vi "edittest export sequence.vi"(6 "User":T1, 8 "error in (no error)":errorcluster, 10 "Sequence ID":string, 11 "Connection Refnum":T2) -> (0 "error out":errorcluster, 2 "Exported Sequence":string, 3 "Connection Refnum":T2)   [LabVIEW 2011]
uses:
  SI.LIB/ODBC/SQL Controls/Connection Refnum.ctl
  server/database/Users/User Record.ctl
  sequence xml.ctl
  server/database/Sequences/Sequence Record.ctl
  server/database/Steps/Step Record.ctl
  server/database/Fields/Field Record.ctl
  server/database/Fields/Field DataTypes.ctl
  server/database/Fields/Field NextItem.ctl
  server/server lib/Spartan Version.vi
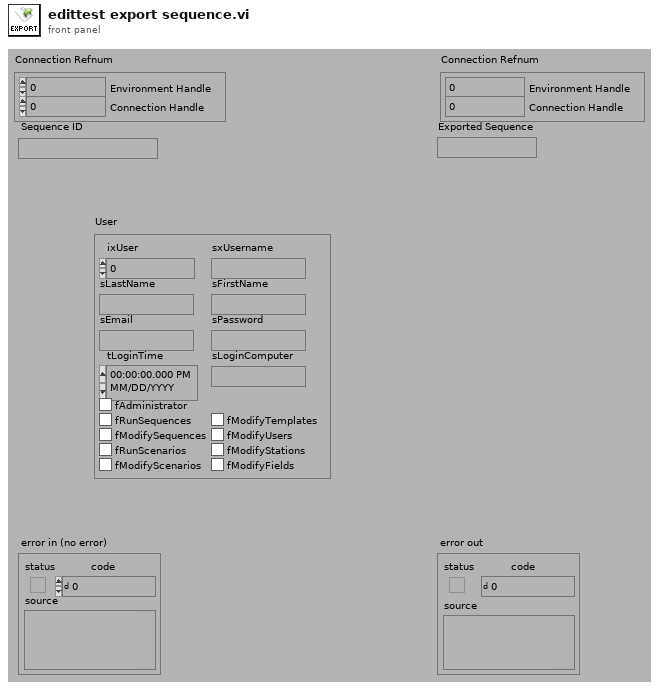
[diagram p1: front panel]
types:
  T1 = typedef "User Record.ctl" = cluster{"ixUser":i32, "sxUsername":string, "sLastName":string, "sFirstName":string, "sEmail":string, "sPassword":string, "tLoginTime":timestamp, "sLoginComputer":string, "fAdministrator":bool, "fRunSequences":bool, "fModifySequences":bool, "fRunScenarios":bool, "fModifyScenarios":bool, "fModifyTemplates":bool, "fModifyUsers":bool, "fModifyStations":bool, "fModifyFields":bool}
  T2 = typedef "Connection Refnum.ctl" = cluster{"Environment Handle":i32, "Connection Handle":i32}
  T3 = typedef "sequence xml.ctl" = cluster{"#attributes":cluster{"Version":string, "Creator":string}, "Sequence":T4, "Steps":T5[], "Fields":T6[]}
  T4 = typedef "Sequence Record.ctl" = cluster{"ixSequence":i32, "sxSequenceId":string, "sDescription":string, "sCreator":string, "tCreationDate":timestamp, "sModifier":string, "tModifiedDate":timestamp, "fApproved":bool, "fSpartanSetsSN":bool, "fOverwriteData":bool, "fStopOnFail":bool, "fDisableQuickMode":bool, "fPartialExecution":bool, "fAutoNextItem":bool, "fDoNotPrintOnFail":bool}
  T5 = typedef "Step Record.ctl" = cluster{"ixStep":i32, "sxSequenceId":string, "sxTestId":string, "iIndex":i32, "iRepeat":i32, "iQuickMode":i32, "sTag":string, "sDatasheetsCSV":string, "bConfiguration":string}
  T6 = typedef "Field Record.ctl" = cluster{"ixField":i32, "iSequenceOrder":i32, "sxFieldId":string, "sxSequenceId":string, "sDisplayName":string, "sValue":string, "sUnits":string, "nDataType":T7, "nNextItem":T8, "fSystem":bool, "fSystemValue":bool, "fRequired":bool, "fSetAtTest":bool, "fTestField":bool, "fDeleted":bool, "fIndexed":bool, "fFreeList":bool}
  T7 = typedef "Field DataTypes.ctl" = enum32{"text", "numeric", "list", "timestamp", "boolean"}
  T8 = typedef "Field NextItem.ctl" = enum32{"Reset", "Retain", "Auto-Increment"}
  T9 = typedef "OGAB Version.ctl" = cluster{"Version":string, "Build Number":u32, "Build Date/Time":dbl}
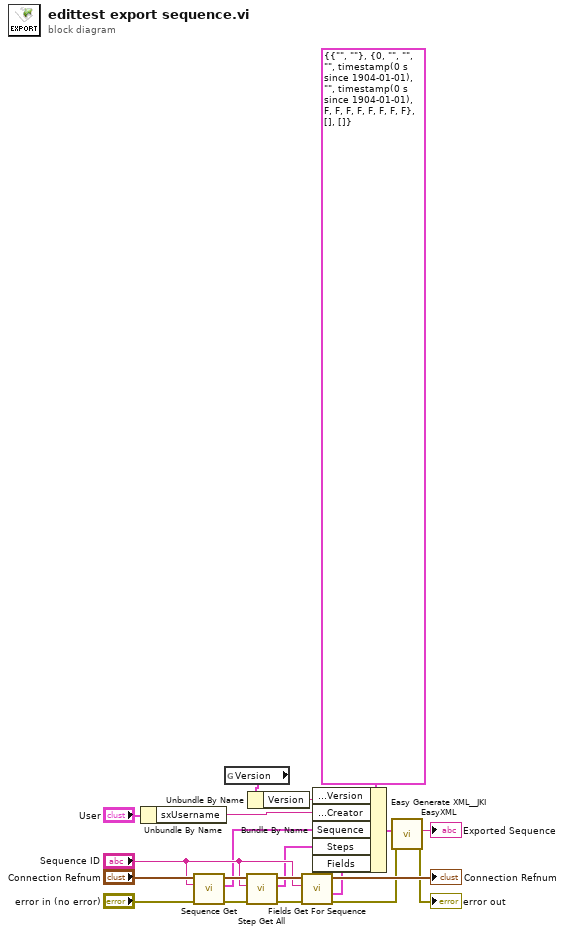
[diagram p0: block diagram]
diagram:
  n1 = Unbundle By Name("User") -> ("sxUsername"=w8:string)
  n2 = call "Sequence Get.vi"("error in (no error)"="error in (no error)", "sxSequenceId (\"\")"="Sequence ID", "Connection Refnum"="Connection Refnum") -> ("error out"=w19:errorcluster, "Sequence Record"=w7:T4, "Connection Refnum"=w16:T2)  [unwired: 6 out]
  n3 = global read "Spartan Version.vi" "Version"() -> (w10:T9)
  n4 = call "Step Get All.vi"("error in (no error)"=w19, "sxSequenceId"="Sequence ID", "Connection Refnum"=w16) -> ("error out"=w17:errorcluster, "Sequence Steps"=w6:T5[], "Connection Refnum"=w15:T2)  [unwired: 1 in, 5 out]
  n5 = Unbundle By Name(w10) -> ("Version"=w9:string)
  n6 = call "Fields Get For Sequence.vi"("error in (no error)"=w17, "sxSequenceId (\"\")"="Sequence ID", "Connection Refnum"=w15) -> ("error out"=w3:errorcluster, "Current Sequence Fields"=w5:T6[], "Connection Refnum"=→"Connection Refnum":T2)  [unwired: 6 out]
  n7 = Bundle By Name(cluster=T3 {"#attributes"={"Version"="", "Creator"=""}, "Sequence"={"ixSequence"=0, "sxSequenceId"="", "sDescription"="", "sCreator"="", "tCreationDate"=timestamp(0 s since 1904-01-01), "sModifier"="", "tModifiedDate"=timestamp(0 s since 1904-01-01), "fApproved"=FALSE, "fSpartanSetsSN"=FALSE, "fOverwriteData"=FALSE, "fStopOnFail"=FALSE, "fDisableQuickMode"=FALSE, "fPartialExecution"=FALSE, "fAutoNextItem"=FALSE, "fDoNotPrintOnFail"=FALSE}, "Steps"=[], "Fields"=[]} ("Sequence"), "#attributes.Version"=w9, "#attributes.Creator"=w8, "Sequence"=w7, "Steps"=w6, "Fields"=w5) -> (w4:T3)
  n8 = call "Easy Generate XML__JKI EasyXML.vi"("error in (no error)"=w3, "LabVIEW Data"=w4) -> ("error out"=→"error out":errorcluster, "XML String"=→"Exported Sequence":string)  [unwired: 8 out]
